vi "Get Classes Names.vi"() -> (3 "Classes":string[](array[string]))   [LabVIEW 2020, in "FGen.lvlib"]
uses:
  FGen.lvlib
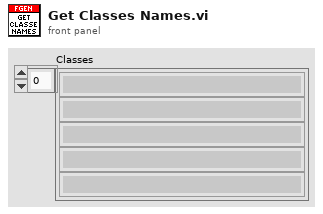
[diagram p1: front panel]
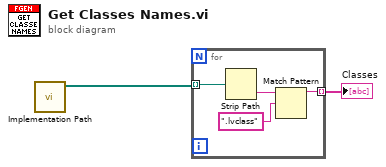
[diagram p0: block diagram]
diagram:
  n1 = call "Implementation Path.vi"() -> ("All Files in Dir"=w1:path[])  [unwired: 11 in]
  n2 = for {
    tunnel: w1 -> [w6] mode=indexing
    tunnel: [w3] -> w2 mode=indexing
    n3 = Strip Path(path=w6) -> (name=w5:string)  [unwired: 1 out]
    n4 = Match Pattern(string=w5, regular expression=".lvclass") -> (before substring=w3:string)  [unwired: 1 in, 3 out]
  }
  "Classes" <- w2
